vi "string to commands.vi"(11 "command string":string) -> (2 "invalid":bool, 3 "commands":T1)   [LabVIEW 2014, in "SMSLD TBD execution service.lvlib"]
uses:
  SMSLD TBD execution service.lvlib
  command commands to rtexe process.ctl
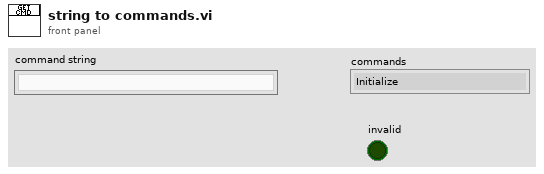
[diagram p1: front panel]
types:
  T1 = typedef "SMSLD TBD execution service.lvlib/command commands to rtexe process.ctl" = enum16{"Initialize", "Add Search Paths", "Load from File", "Unload File", "Open All Engines", "Open Single Engine", "Initialize All Engines", "Initialize Single Engine", "Start All", "Start Single", "Pause All", "Pause Single", "Stop All", "Stop Single", "Close All", "Close Single", "Set Safe State All", "Set Safe State Single", "Get Status", "Exit", "Error", "Load Bitfile", "Unload Bitfile", "Clear Faults Single", "Clear Faults All"}
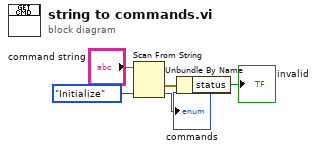
[diagram p0: block diagram]
diagram:
  n1 = Scan From String(input string="command string", default 1=command_commands_to_rtexe_process."Initialize" ("commands")) -> (error out=w2:errorcluster, output 1=→"commands":T1)  [unwired: 3 in, 2 out]
  n2 = Unbundle By Name(w2) -> ("status"=→"invalid":bool)
